vi "Dequeue Message.vi"(7 "Diagnostics Queue":refnum<queue>, 8 "error in (no error)":errorcluster, 11 "Message Queue":refnum<queue>) -> (0 "error out":errorcluster, 1 "Message Data":variant, 2 "Message":string, 3 "dup Message Queue":refnum<queue>)   [LabVIEW 2021, in "Message Queue.lvlib"]
doc: "This VI pulls messages off the Message Queue."
uses:
  Message Queue.lvlib
  Message Cluster.ctl
  Enqueue Message (Single).vi
panel:
  out "elements":T1[](array[typedef])
  out "# pending remove":i32
  out "# pending insert":i32
  out "# elements in queue":i32
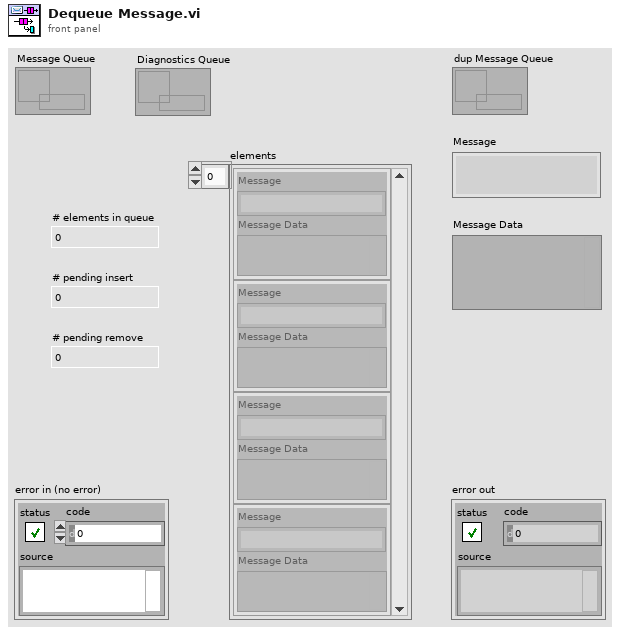
[diagram p1: front panel]
types:
  T1 = typedef "Message Queue.lvlib/Message Cluster.ctl" = cluster{"Message":string, "Message Data":variant}
  T2 = cluster{"Message Cluster":T1, "Call Stack":string[]}
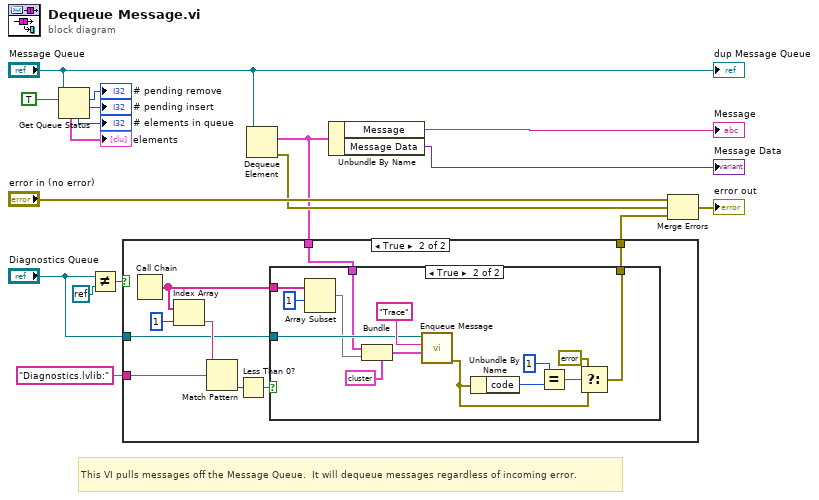
[diagram p0: block diagram]
diagram:
  # "This VI pulls messages off the Message Queue.  It will dequeue messages regardless of incoming error."
  n1 = Get Queue Status(queue="Message Queue", return elements? (F)=TRUE) -> (# pending remove=→"# pending remove":i32, # pending insert=→"# pending insert":i32, # elements in queue=→"# elements in queue":i32, elements=→"elements":T1[])  [unwired: 1 in, 4 out]
  n2 = Not Equal?(x="Diagnostics Queue", y=refnum<k0> refnum) -> (x != y?=w10:bool)
  n3 = Dequeue Element(queue="Message Queue") -> (element=w12:T1, error out=w13:errorcluster)  [unwired: 2 in, 2 out]
  n4 = case shown="True" w10 {
    tunnel: w12 -> [_ w26]
    tunnel: "Diagnostics.lvlib:" -> [_ w24]
    tunnel: "Diagnostics Queue" -> [_ w20]
    tunnel: [_ w18] -> w7
    frame False {
    }
    frame True {
      n5 = Call Chain() -> (call chain=w19:string[])
      n6 = Index Array(array=w19, index=1) -> (element=w22:string)
      n7 = Match Pattern(string=w22, regular expression=w24) -> (offset past match=w25:i32)  [unwired: 1 in, 3 out]
      n8 = Less Than 0?(x=w25) -> (x < 0?=w21:bool)
      n9 = case shown="True" w21 {
        tunnel: w26 -> [_ w36]
        tunnel: w20 -> [_ w39]
        tunnel: w19 -> [_ w38]
        tunnel: [_ w28] -> w18
        frame False {
        }
        frame True {
          n10 = Array Subset(array=w38, index=1) -> (w35:string[])  [unwired: 1 in]
          n11 = Bundle(cluster=T2 {"Message Cluster"={"Message"="", "Message Data"=variant}, "Call Stack"=[]}, "Message Cluster"=w36, "Call Stack"=w35) -> (w34:T2)
          n12 = call-poly "Enqueue Message.vi"("Message Data"=w34, "Message"="Trace", "Message Queue"=w39) -> ("error out"=w27:errorcluster)  [unwired: 7 in, 1 out]
          n13 = Unbundle By Name(w27) -> ("code"=w31:i32)
          n14 = Equal?(x=1, y=w31) -> (x = y?=w32:bool)
          n15 = Select(t=errorcluster {"status"=FALSE, "code"=0, "source"=""} ("No Error"), s=w32, f=w27) -> (s? t:f=w28:errorcluster)
        }
      }
    }
  }
  n16 = Unbundle By Name(w12) -> ("Message"=→"Message":string, "Message Data"=→"Message Data":variant)
  n17 = Merge Errors("error in (no error)", w13, w7) -> (→"error out":errorcluster)
  "dup Message Queue" <- "Message Queue"
